vi "Main.vi"() -> ()   [LabVIEW 2017]
uses:
  Controls/Control 1.ctl
panel:
  in  "Slide":T1 scale=0.0..10.0
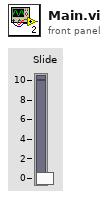
[diagram p1: front panel]
types:
  T1 = typedef "Control 1.ctl" = dbl
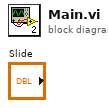
[diagram p0: block diagram]
diagram:
